vi "string to Connection.vi"(10 "String":string) -> (2 "connections":T1)   [LabVIEW 2015, in "SLSC Switch.lvclass"]
uses:
  SLSC Switch/SLSC Switch.lvclass
  SLSC Switch/Controls/Connection.ctl
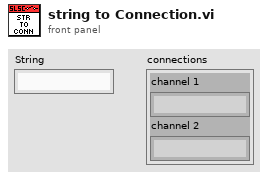
[diagram p1: front panel]
types:
  T1 = typedef "SLSC Switch.lvclass/Connection.ctl" = cluster{"channel 1":string, "channel 2":string}
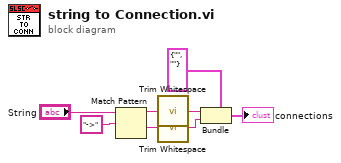
[diagram p0: block diagram]
diagram:
  n1 = Match Pattern(string="String", regular expression="->") -> (before substring=w6:string, after substring=w5:string)  [unwired: 1 in, 2 out]
  n2 = call <vilib>:"Trim Whitespace.vi"("string"=w6) -> ("trimmed string"=w3:string)  [unwired: 1 in]
  n3 = call <vilib>:"Trim Whitespace.vi"("string"=w5) -> ("trimmed string"=w2:string)  [unwired: 1 in]
  n4 = Bundle(cluster=T1 {"channel 1"="", "channel 2"=""} ("connections"), "channel 1"=w3, "channel 2"=w2) -> (→"connections":T1)
